vi "Get Class Object.vi"(8 "error in (no error)":errorcluster, 11 "Parent Value":bool) -> (0 "error out":errorcluster, 3 "class string":refnum<class "Parent.lvclass">)   [LabVIEW 2023]
doc: "Gets the string data from Parent.lvclass or Child.lvclass, depending on <B>Parent Value</B>. When <B>Parent Value</B> is <B>True</B>, this VI calls the Write String Data VI of Parent.lvclass to get the string data. Otherwise, this VI calls the Write String VI of Child.lvclass to get the string data.\nUse this VI as a setup VI for the Dynamic Dispatch Method.lvtest."
uses:
  Parent/Parent.lvclass
  Child.lvclass
  c:/dev/_r/36/eng/lv-modules-toolkits/toolkits/utf_lv_support/objects/lv/win32U/examples/Unit Test Framework/LabVIEW Class/Parent/Parent.lvclass
panel:
  # "Overview: Gets the string data from Parent.lvclass or Child.lvclass, depending on Parent Value. Use this VI as a setup VI for the Dynamic Dispatch Method.lvtest."
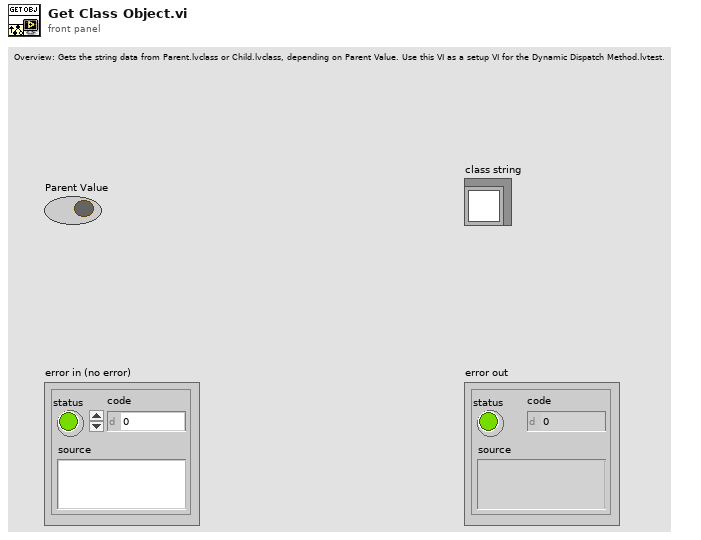
[diagram p1: front panel]
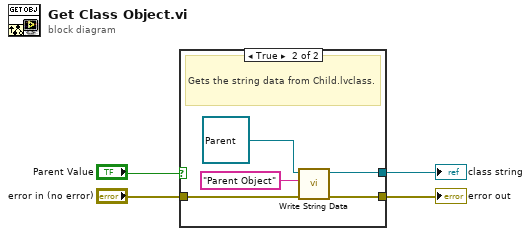
[diagram p0: block diagram]
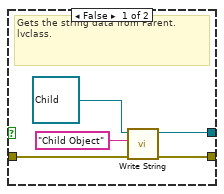
[diagram p2: hidden frame]
diagram:
  n1 = case shown="True" "Parent Value" {
    tunnel: [w8 w13] -> w4
    tunnel: "error in (no error)" -> [w6 w11]
    tunnel: [w7 w10] -> w1
    frame False {
      # "Gets the string data from Parent.lvclass."
      n2 = call "Write String.vi"("error in (no error)"=w6, "String"="Child Object", "class string child in"=refnum<class "Child.lvclass"> refnum ("clsStringChild.lvclass")) -> ("error out"=w7:errorcluster, "class string child out"=w8:refnum<class "Child.lvclass">)  [unwired: 7 in]
    }
    frame True {
      # "Gets the string data from Child.lvclass."
      n3 = call-dynamic "Write String Data.vi"("error in (no error)"=w11, "String Data"="Parent Object" ("String"), "class string in"=refnum<class "Parent.lvclass"> refnum ("clsString.lvclass")) -> ("error out"=w10:errorcluster, "class string out"=w13:refnum<class "Parent.lvclass">)  [unwired: 7 in]
    }
  }
  "class string" <- w4
  "error out" <- w1
